vi "Triax320 GetParams.vi"(8 "error in":errorcluster, 10 "Grating":u8(ring) items=["1", "2", "3"], 11 "Param":T1=enum."Tous") -> (0 "error out":errorcluster, 1 "LineDensity":u32 caption="Line Density\n(Groove/mm)", 2 "CalOffset":i32=-1641 caption="Cal Offset", 4 "OutSlit":dbl=0.01 caption="Output Slit(mm)" format="%#_7g", 5 "Grating Description":string, 6 "InSlit":dbl=0.01 caption="Input Slit(mm)" format="%#_7g")   [LabVIEW 2019]
doc: "Ce Vi enregistre les paramètres des différents axes dans un fichier .ini"
uses:
  <userlib>/Triax320/TriaxParams.ctl
  <vilib>/Utility/config.llb/Read Key (U32).vi
  <vilib>/Utility/config.llb/Read Key (I32).vi
  <vilib>/Utility/config.llb/Read Key (Double).vi
  <vilib>/Utility/config.llb/Read Key (String).vi
  <vilib>/Utility/config.llb/NI_LVConfig.lvlib
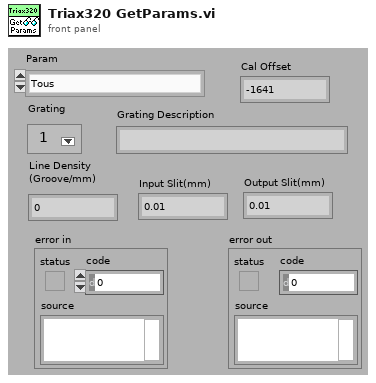
[diagram p1: front panel]
types:
  T1 = typedef "TriaxParams.ctl" = enum16{"Grating", "CalOffset", "Line Density (grv/mm)", "Input Slit (mm)", "Output Slit (mm)", "Both Slit (mm)", "Grating Desc.", "Tous"}
  T2 = typedef "NI_LVConfig.lvlib/Config Data RefNum.ctl" = refnum<k1>
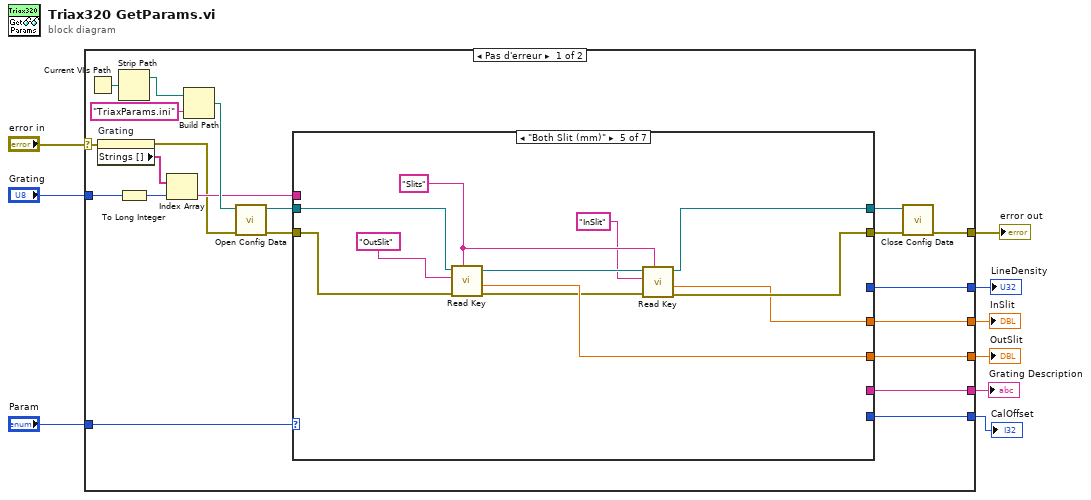
[diagram p0: block diagram]
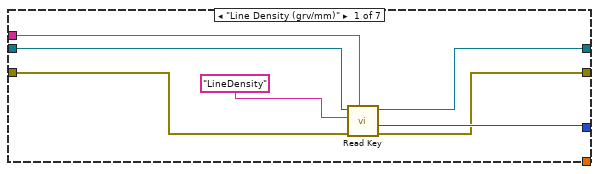
[diagram p2: hidden frame]
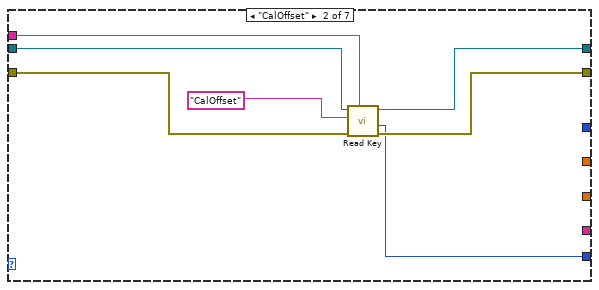
[diagram p3: hidden frame]
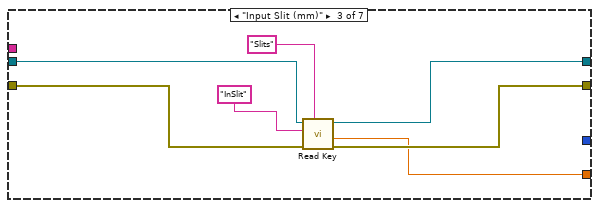
[diagram p4: hidden frame]
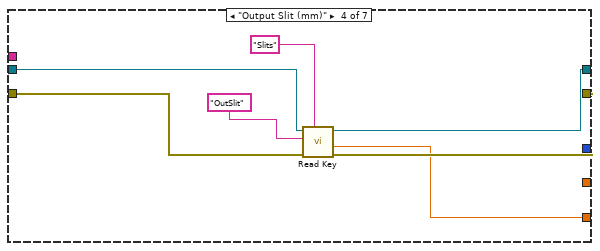
[diagram p5: hidden frame]
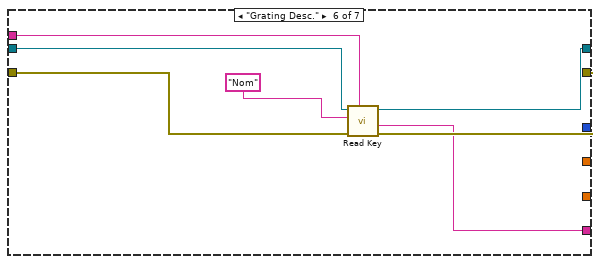
[diagram p6: hidden frame]
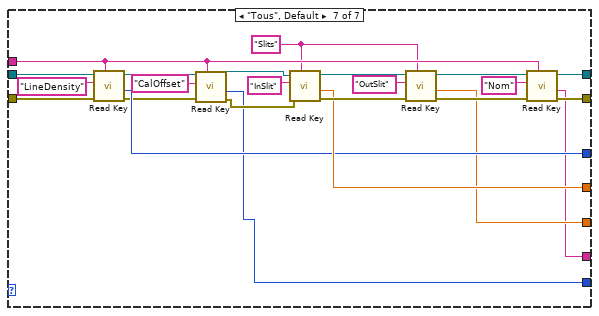
[diagram p7: hidden frame]
diagram:
  n1 = case shown="Pas d'erreur" "error in" {
    selector: "error in" -> [w17 w101]
    tunnel: "Grating" -> [w27 _]
    tunnel: [w23 w101] -> w8
    tunnel: "Param" -> [w19 _]
    tunnel: [w14 _] -> w5
    tunnel: [w13 _] -> w4
    tunnel: [w12 _] -> w3
    tunnel: [w11 _] -> w2
    tunnel: [w10 _] -> w1
    frame No Error {
      n2 = Current VI's Path() -> (path=w30:path)
      n3 = property on="Grating" class="MDér (strict)"(error in=w17) -> (error out=w16:errorcluster, "Strings []"=w26:string[])  [unwired: 1 in, 1 out]
      n4 = Strip Path(path=w30) -> (stripped path=w18:path)  [unwired: 1 out]
      n5 = To Long Integer(number=w27) -> (32bit integer=w15:i32)
      n6 = Index Array(array=w26, index=w15) -> (element=w22:string)
      n7 = Build Path(base path=w18, name or relative path="TriaxParams.ini") -> (appended path=w28:path)
      n8 = call <vilib>:"Open Config Data.vi"("error in (no error)"=w16, "configuration file path"=w28) -> ("error out"=w24:errorcluster, "refnum"=w25:T2)  [unwired: 7 in, 1 out]
      n9 = case shown="\"Both Slit (mm)\"" w19 {
        tunnel: w25 -> [w35 w42 w50 w56 w69 w73 w90]
        tunnel: w24 -> [w34 w41 w49 w55 w68 w72 w89]
        tunnel: w22 -> [w37 w44 _ _ _ w76 w78]
        tunnel: [w31 w40 w47 w58 w62 w75 w91] -> w21
        tunnel: [w36 w43 w51 w57 w61 w74 w92] -> w20
        tunnel: [_ _ w46 _ w60 _ w88] -> w14
        tunnel: [w32 _ _ _ _ _ w87] -> w13
        tunnel: [_ _ _ w53 w66 _ w86] -> w12
        tunnel: [_ _ _ _ _ w70 w85] -> w11
        tunnel: [_ w38 _ _ _ _ w79] -> w10
        frame "Line Density (grv/mm)" {
          n10 = call-poly <vilib>:"Read Key.vi"("section"=w37, "error in (no error)"=w34, "key"="LineDensity", "refnum"=w35) -> ("error out"=w31:errorcluster, "value"=w32:u32, "refnum out"=w36:T2)  [unwired: 4 in, 1 out]
        }
        frame "CalOffset" {
          n11 = call-poly <vilib>:"Read Key.vi"("section"=w44, "error in (no error)"=w41, "key"="CalOffset", "refnum"=w42) -> ("error out"=w40:errorcluster, "value"=w38:i32, "refnum out"=w43:T2)  [unwired: 4 in, 1 out]
        }
        frame "Input Slit (mm)" {
          n12 = call-poly <vilib>:"Read Key.vi"("section"="Slits", "error in (no error)"=w49, "key"="InSlit", "refnum"=w50) -> ("error out"=w47:errorcluster, "value"=w46:dbl, "refnum out"=w51:T2)  [unwired: 4 in, 1 out]
        }
        frame "Output Slit (mm)" {
          n13 = call-poly <vilib>:"Read Key.vi"("section"="Slits", "error in (no error)"=w55, "key"="OutSlit", "refnum"=w56) -> ("error out"=w58:errorcluster, "value"=w53:dbl, "refnum out"=w57:T2)  [unwired: 4 in, 1 out]
        }
        frame "Both Slit (mm)" {
          w65 = "Slits" ("section")
          n14 = call-poly <vilib>:"Read Key.vi"("section"=w65, "error in (no error)"=w68, "key"="OutSlit", "refnum"=w69) -> ("error out"=w63:errorcluster, "value"=w66:dbl, "refnum out"=w64:T2)  [unwired: 4 in, 1 out]
          n15 = call-poly <vilib>:"Read Key.vi"("section"=w65, "error in (no error)"=w63, "key"="InSlit", "refnum"=w64) -> ("error out"=w62:errorcluster, "value"=w60:dbl, "refnum out"=w61:T2)  [unwired: 4 in, 1 out]
        }
        frame "Grating Desc." {
          n16 = call-poly <vilib>:"Read Key.vi"("section"=w76, "error in (no error)"=w72, "key"="Nom", "refnum"=w73) -> ("error out"=w75:errorcluster, "value"=w70:string, "refnum out"=w74:T2)  [unwired: 4 in, 1 out]
        }
        frame "Tous", Default {
          w77 = "Slits" ("section")
          n17 = call-poly <vilib>:"Read Key.vi"("section"=w78, "error in (no error)"=w89, "key"="LineDensity", "refnum"=w90) -> ("error out"=w84:errorcluster, "value"=w87:u32, "refnum out"=w82:T2)  [unwired: 4 in, 1 out]
          n18 = call-poly <vilib>:"Read Key.vi"("section"=w78, "error in (no error)"=w84, "key"="CalOffset", "refnum"=w82) -> ("error out"=w83:errorcluster, "value"=w79:i32, "refnum out"=w81:T2)  [unwired: 4 in, 1 out]
          n19 = call-poly <vilib>:"Read Key.vi"("section"=w77, "error in (no error)"=w83, "key"="InSlit", "refnum"=w81) -> ("error out"=w96:errorcluster, "value"=w88:dbl, "refnum out"=w93:T2)  [unwired: 4 in, 1 out]
          n20 = call-poly <vilib>:"Read Key.vi"("section"=w77, "error in (no error)"=w96, "key"="OutSlit", "refnum"=w93) -> ("error out"=w95:errorcluster, "value"=w86:dbl, "refnum out"=w94:T2)  [unwired: 4 in, 1 out]
          n21 = call-poly <vilib>:"Read Key.vi"("section"=w78, "error in (no error)"=w95, "key"="Nom", "refnum"=w94) -> ("error out"=w91:errorcluster, "value"=w85:string, "refnum out"=w92:T2)  [unwired: 4 in, 1 out]
        }
      }
      n22 = call <vilib>:"Close Config Data.vi"("error in (no error)"=w21, "refnum"=w20) -> ("error out"=w23:errorcluster)  [unwired: 8 in, 1 out]
    }
    frame Error {
    }
  }
  "error out" <- w8
  "Grating Description" <- w2
  "LineDensity" <- w4
  "InSlit" <- w5
  "OutSlit" <- w3
  "CalOffset" <- w1
